vi "run_autoProtocol_v02.vi"(6 "control label":string, 8 "error in":errorcluster, 9 "data in":T1={"daq_ao 1"="Dev1/ao0", "daq_ai 1"="Dev1/ai0", "experiment day folder"=path "D:/DATA/8-27-15 save func testing/test.lvm", "Multiclamp init error"=0, "Multiclamp Handle Out"=0, "sampling rate (Hz)"=10000, "trial name"=""}, 10 "clamp switch (T=v, F=i)":bool, 11 "controls array":refnum<vi>[](array[refnum])) -> (0 "error out":errorcluster, 1 "data out":T1={"daq_ao 1"="Dev1/ao0", "daq_ai 1"="Dev1/ai0", "experiment day folder"=path "D:/DATA/8-27-15 save func testing/test.lvm", "Multiclamp init error"=0, "Multiclamp Handle Out"=0, "sampling rate (Hz)"=10000, "trial name"=""}, 3 "controls array out":refnum<vi>[](array[refnum]))   [LabVIEW 2015]
uses:
  get_data_from_control_prot.vi
  Controls/Data.ctl
panel:
  out "View profile (wvfrms)":waveform(dbl)[](graph)
  # "RUN_AUTOPROTOCOL"
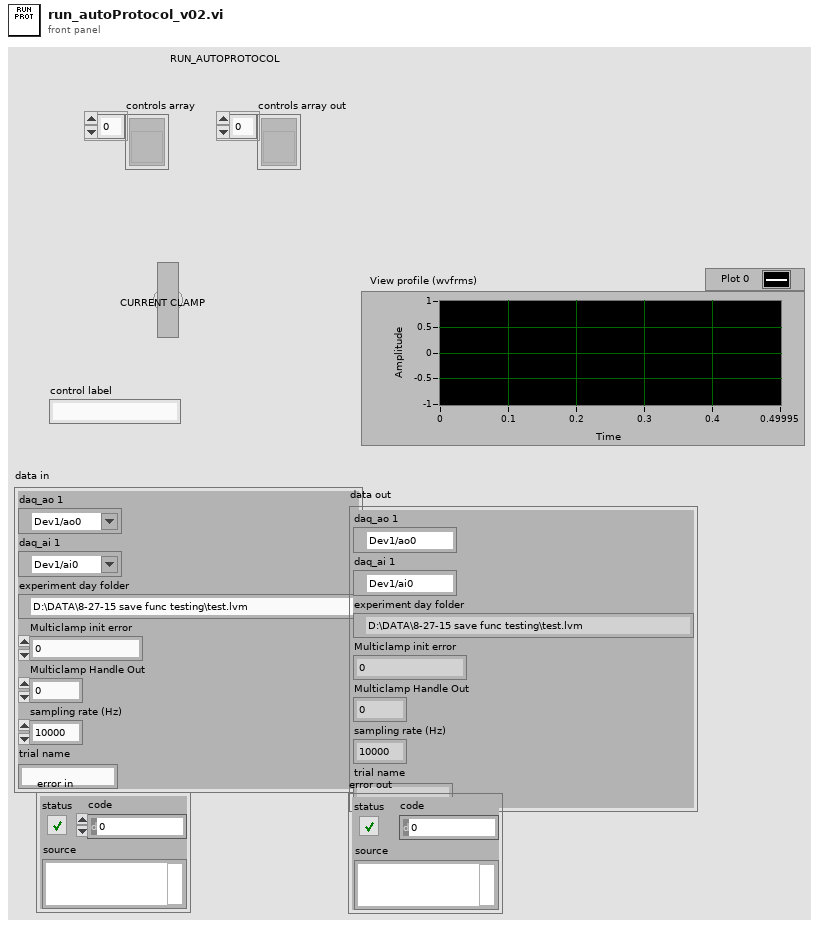
[diagram p1: front panel]
types:
  T1 = typedef "Data.ctl" = cluster{"daq_ao 1":tag, "daq_ai 1":tag, "experiment day folder":path, "Multiclamp init error":i32, "Multiclamp Handle Out":u32, "sampling rate (Hz)":i32, "trial name":string}
  T2 = typedef "clamp_profile.ctl" = cluster{"aLevel":dbl, "aDelta":dbl, "aDuration":i32, "bLevel":dbl, "bDelta":dbl, "bDuration":i32, "cLevel":dbl, "cDelta":dbl, "cDuration":i32}
  T3 = cluster{"Iclamp in":T2, "# iter":i32, "# reps IC":i32}
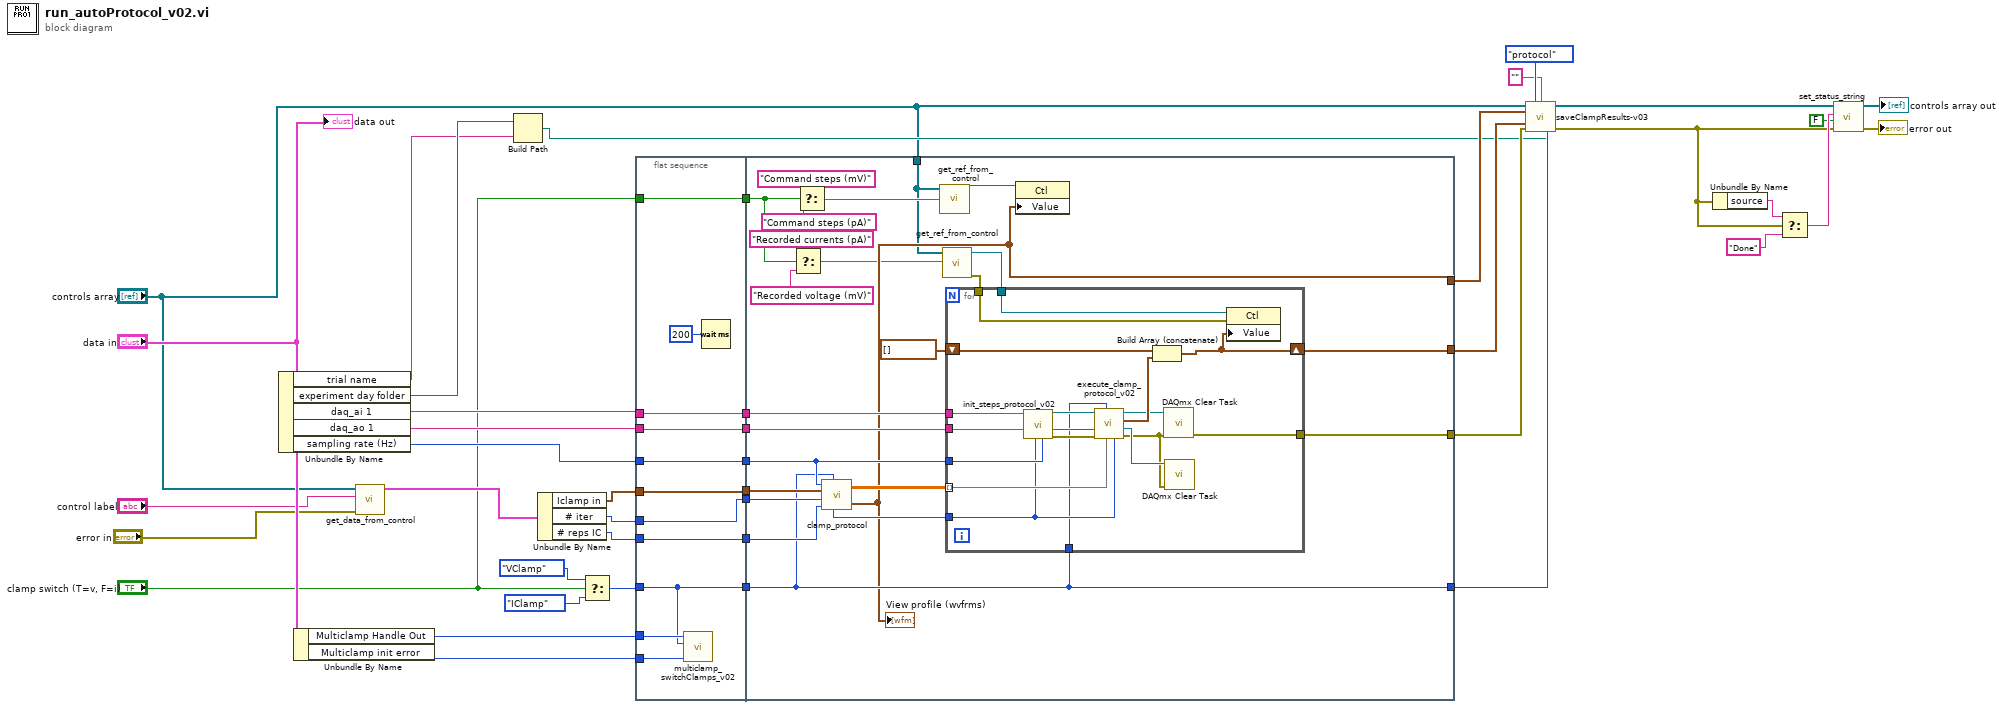
[diagram p0: block diagram]
diagram:
  n1 = Unbundle By Name("data in") -> ("trial name"=w6:string, "experiment day folder"=w7:path, "daq_ai 1"=w27:tag, "daq_ao 1"=w26:tag, "sampling rate (Hz)"=w25:i32)
  n2 = Unbundle By Name("data in") -> ("Multiclamp Handle Out"=w23:u32, "Multiclamp init error"=w22:i32)
  n3 = call-poly "get_data_from_control.vi"("error in"="error in", "control label"="control label", "controls array"="controls array") -> ("Prot output"=w17:T3)  [unwired: 7 in, 1 out]
  n4 = Build Path(base path=w7, name or relative path=w6) -> (appended path=w3:path)
  n5 = Unbundle By Name(w17) -> ("Iclamp in"=w21:T2, "# iter"=w20:i32, "# reps IC"=w19:i32)
  n6 = Select(t=enum16{"VClamp", "IClamp"}."VClamp" ("which clamp"), s="clamp switch (T=v, F=i)", f=enum16{"VClamp", "IClamp"}."IClamp" ("which clamp")) -> (s? t:f=w40:enum16{"VClamp", "IClamp"})
  n7 = flat-sequence {
    tunnel: w23 -> [w52]
    tunnel: w22 -> [w51]
    tunnel: w40 -> [w46]
    tunnel: w20 -> [w50]
    tunnel: [w50] -> w39
    tunnel: w19 -> [w49]
    tunnel: [w49] -> w38
    tunnel: w21 -> [w48]
    tunnel: [w48] -> w37
    tunnel: w25 -> [w47]
    tunnel: [w47] -> w36
    tunnel: [w46] -> w35
    tunnel: [w45] -> w34
    tunnel: w27 -> [w45]
    tunnel: w26 -> [w44]
    tunnel: [w44] -> w33
    tunnel: "clamp switch (T=v, F=i)" -> [w43]
    tunnel: [w43] -> w8
    tunnel: w39 -> [w76]
    tunnel: w38 -> [w75]
    tunnel: w37 -> [w74]
    tunnel: w36 -> [w71]
    tunnel: w35 -> [w66]
    tunnel: w34 -> [w73]
    tunnel: w33 -> [w72]
    tunnel: [w68] -> w31
    tunnel: [w61] -> w32
    tunnel: [w67] -> w30
    tunnel: [w66] -> w28
    tunnel: "controls array" -> [w60]
    tunnel: w8 -> [w55]
    frame #0 {
      n8 = call "multiclamp_switchClamps_v02.vi"("error in"=w51, "which clamp"=w46, "Multiclamp Handle in"=w52) -> ()  [unwired: 7 in, 2 out]
      n9 = Wait (ms)(milliseconds to wait=u32 200) -> ()  [unwired: 1 out]
    }
    frame #1 {
      n10 = Select(t="Recorded currents (pA)", s=w55, f="Recorded voltage (mV)") -> (s? t:f=w59:string)
      n11 = Select(t="Command steps (mV)", s=w55, f="Command steps (pA)") -> (s? t:f=w63:string)
      n12 = call "clamp_protocol.vi"("which clamp"=w66, "# reps"=w75, "# Iterations"=w76, "clamp in"=w74, "sampling rate (Hz)"=w71) -> ("View profile (wvfrms)"=w61:waveform(dbl)[], "Stim profile"=w70:dbl[][], "samples to read"=w77:i32)
      "View profile (wvfrms)" <- w61
      n13 = call "get_ref_from_control.vi"("control label"=w63, "controls array"=w60) -> ("reference out"=w62:refnum<vi>)  [unwired: 8 in, 1 out]
      n14 = call "get_ref_from_control.vi"("control label"=w59, "controls array"=w60) -> ("error out"=w56:errorcluster, "reference out"=w57:refnum<vi>)  [unwired: 8 in]
      n15 = for {
        tunnel: w77 -> [w91]
        tunnel: w73 -> [w95]
        tunnel: w72 -> [w94]
        tunnel: w71 -> [w93]
        tunnel: w70 -> [w92] mode=indexing
        tunnel: w66 -> [w87]
        shift-right: [w78] -> w68
        shift-left: waveform(dbl)[] [] -> [w85]
        tunnel: [w81] -> w67
        tunnel: w57 -> [w80]
        tunnel: w56 -> [w79]
        n16 = call "init_steps_protocol_v02.vi"("sampling rate (Hz)"=w93, "samples to read"=w91, "AO physical channels"=w94, "AI Physical Channel"=w95) -> ("error out"=w88:errorcluster, "AO out"=w89:refnum<k21>, "AI out"=w90:refnum<k21>)  [unwired: 5 in]
        n17 = call "execute_clamp_protocol_v02.vi"("number of samples per channel"=w91, "command data in"=w92, "which clamp"=w87, "error in"=w88, "AO in"=w89, "AI in"=w90) -> ("error out"=w82:errorcluster, "AO out"=w83:refnum<k21>, "output Graph"=w86:waveform(dbl), "AI out"=w84:refnum<k21>)  [unwired: 2 in]
        n18 = Build Array (concatenate)(w85, w86) -> (w78:waveform(dbl)[])
        n19 = call <vilib>:"DAQmx Clear Task.vi"("task in"=w84, "error in"=w82) -> ("error out"=w81:errorcluster)  [unwired: 13 in]
        n20 = call <vilib>:"DAQmx Clear Task.vi"("task in"=w83, "error in"=w82) -> ()  [unwired: 13 in, 1 out]
        n21 = property class="Ctl"(reference=w80, error in=w79, "Value"=w78) -> ()  [unwired: 2 out]
      }
      n22 = property class="Ctl"(reference=w62, "Value"=w61) -> ()  [unwired: 1 in, 2 out]
    }
  }
  n23 = call "saveClampResults-v03.vi"("controls array"="controls array", "protocol or memtest"=enum16{"protocol", "memtest"}."protocol", "ExpPhase"="", "which clamp"=w28, "view profile"=w32, "rec profile"=w31, "error in"=w30, "Save to (folder dir)"=w3) -> ("controls array out"=w5:refnum<vi>[], "error out"=w12:errorcluster)  [unwired: 6 in]
  n24 = Unbundle By Name(w12) -> ("source"=w14:string)
  n25 = Select(t=w14, s=w12, f="Done") -> (s? t:f=w15:string)
  n26 = call "set_status_string.vi"("error in"=w12, "new line?"=FALSE, "status string in"=w15, "controls array"=w5) -> ("error out"=→"error out":errorcluster, "controls array out"=→"controls array out":refnum<vi>[])  [unwired: 6 in]
  "data out" <- "data in"
